vi "WTYK_AMC_Framwork.vi"() -> ()   [LabVIEW 2016]
uses:
  <userlib>/WTYK_AMC_Framwork/QueueAct.ctl
panel:
  in  "?":T1
  in  "elements 2":cluster{"State":string, "Data":variant}[](array[cluster])
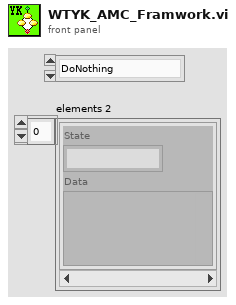
[diagram p1: front panel]
types:
  T1 = typedef "QueueAct.ctl" = enum16{"DoNothing", "AddAfter", "AddBefore", "DeleteOne", "Clear"}
  T2 = enum32{"Invalid", "Standard", "Closed", "Hidden", "Minimized", "Maximized"}
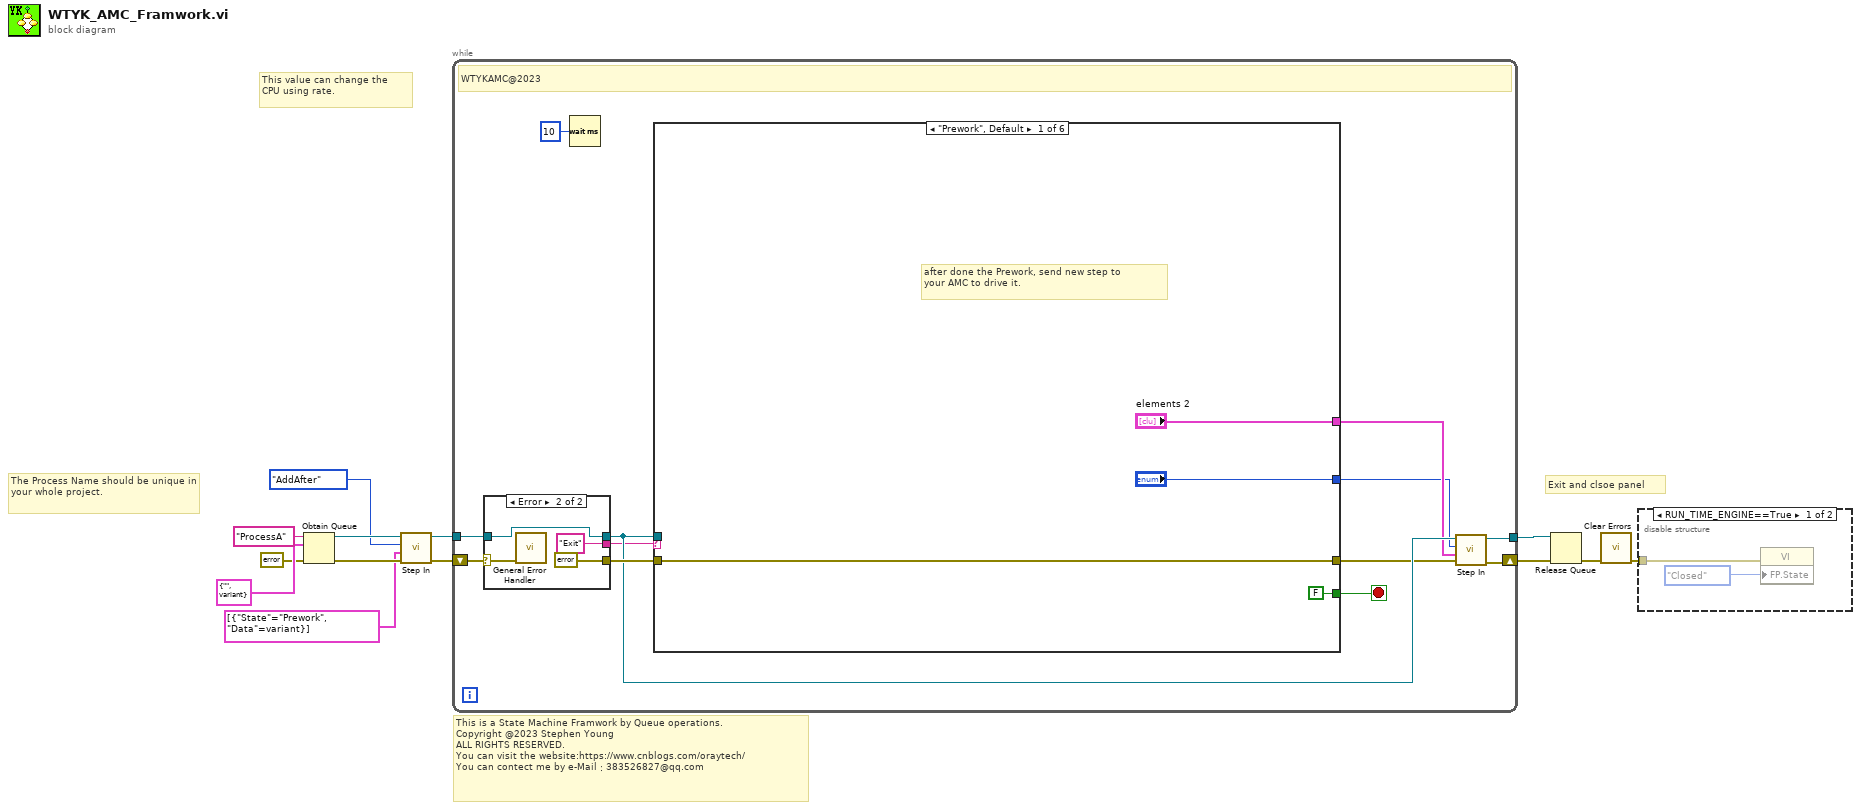
[diagram p0: block diagram]
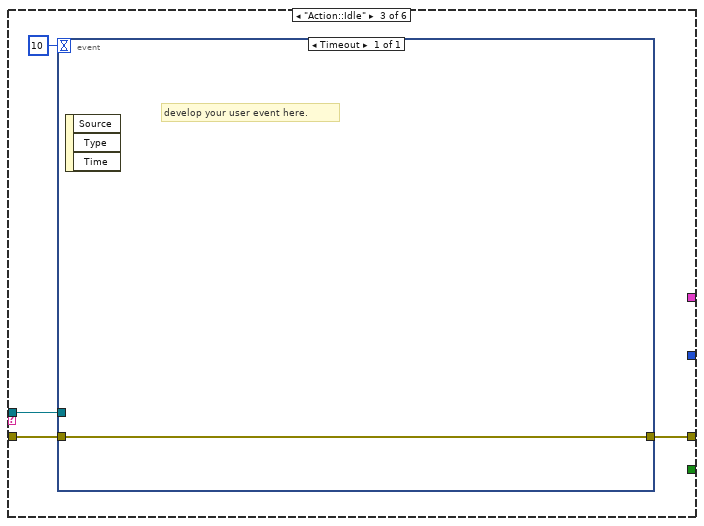
[diagram p4: hidden frame]
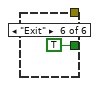
[diagram p7: hidden frame]
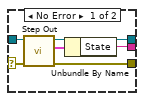
[diagram p8: hidden frame]
diagram:
  # "This is a State Machine Framwork by Queue operations.\nCopyright @2023 Stephen Young \nALL RIGHTS RESERVED.\nYou can visit the website:https://www.cnblogs.com/oraytech/\nYou can contect me by e-Mail：383526827@qq.com"
  # "Exit and clsoe panel"
  # "The Process Name should be unique in your whole project."
  # "This value can change the\nCPU using rate."
  n1 = Obtain Queue(name (unnamed)="ProcessA", element data type=cluster{"State":string, "Data":variant} {"State"="", "Data"=variant}, error in (no error)=errorcluster {"status"=FALSE, "code"=0, "source"=""}) -> (queue out=w6:refnum<queue>, error out=w5:errorcluster)  [unwired: 2 in, 1 out]
  n2 = call <userlib>:"Step In.vi"("error in (no error)"=w5, "elements"=cluster{"State":string, "Data":variant}[] [{"State"="Prework", "Data"=variant}], 10:QueueAct."AddAfter", "QUEUE in"=w6) -> ("error out"=w1:errorcluster, "queue out"=w2:refnum<queue>)  [unwired: 6 in]
  n3 = while {
    shift-right: [w19] -> w11
    shift-left: w1 -> [w25]
    tunnel: [w21] -> w10
    tunnel: w2 -> [w17]
    stop <- w23 stop-if-true
    # "WTYKAMC@2023"
    n4 = case shown="Error" w25 {
      selector: w25 -> [w41 w45]
      tunnel: [w37 "Exit" ("State")] -> w18
      tunnel: [w39 errorcluster {"status"=FALSE, "code"=0, "source"=""} ("error in (no error)")] -> w24
      tunnel: [w38 w42] -> w22
      tunnel: w17 -> [w36 w42]
      frame No Error {
        n5 = call <userlib>:"Step Out.vi"("error in (no error)"=w41, "QUEUE in"=w36) -> ("error out"=w39:errorcluster, "element"=w40:cluster{"State":string, "Data":variant}, "queue out"=w38:refnum<queue>)  [unwired: 6 in, 1 out]
        n6 = Unbundle By Name(w40) -> ("State"=w37:string)
      }
      frame Error {
        n7 = call <vilib>:"General Error Handler.vi"("error in (no error)"=w45) -> ()  [unwired: 2 in, 13 out]
      }
    }
    n8 = Wait (ms)(milliseconds to wait=u32 10) -> ()  [unwired: 1 out]
    n9 = case shown="\"Prework\", Default" w18 {
      tunnel: w24 -> [w29 _ w33 _ _ _]
      tunnel: [w29 _ w32 _ _ _] -> w20
      tunnel: w22 -> [_ _ w31 _ _ _]
      tunnel: [FALSE _ _ _ _ TRUE] -> w23
      tunnel: ["elements 2" _ _ _ _ _] -> w16
      tunnel: ["?" _ _ _ _ _] -> w15
      frame "Prework", Default {
        # "after done the Prework, send new step to\nyour AMC to drive it."
      }
      frame "------Action------" {
      }
      frame "Action::Idle" {
        n10 = event shown="[0] Timeout" {
          selector: _ -> [_]
          dyn-events: _ -> [_]
          timeout: 10 -> [_]
          tunnel: w33 -> [w34]
          tunnel: [w34] -> w32
          tunnel: w31 -> [_]
          event Timeout {
            # "develop your user event here."
            n11 = event-data() -> ()  [unwired: 1 in, 3 out]
          }
        }
      }
      frame "Action::action1" {
        # "Develop your code here"
      }
      frame "------Exit------" {
      }
      frame "Exit" {
      }
    }
    n12 = call <userlib>:"Step In.vi"("error in (no error)"=w20, "elements"=w16, 10:w15, "QUEUE in"=w22) -> ("error out"=w19:errorcluster, "queue out"=w21:refnum<queue>)  [unwired: 6 in]
  }
  n13 = Release Queue(queue=w10, error in (no error)=w11) -> (error out=w9:errorcluster)  [unwired: 3 out]
  n14 = call <vilib>:"Clear Errors.vi"("error in (no error)"=w9) -> ("error out"=w8:errorcluster)  [unwired: 5 in, 1 out]
  n15 = disable-structure shown="RUN_TIME_ENGINE==True" {
    disable-tunnel: w8 -> [w47 _]
    frame condition #0 {
      n16 = property class="VI"(error in=w47, "FP.State"=T2."Closed" ("Front Panel Window:State")) -> ()  [unwired: 1 in, 2 out]
    }
    frame condition #1 (active) {
    }
  }
